vi "Initialize Millisecond Tick Timer Q.vi"(8 "error in (no error)":errorcluster, 11 "DbgTimers in":refnum<class "DbgTimers.lvclass">) -> (0 "error out":errorcluster, 3 "DbgTimers out":refnum<class "DbgTimers.lvclass">)   [LabVIEW 2017, in "DbgTimers.lvclass"]
doc: "Developed by Kevin Thompson\nkevin@thompsonengineering.net\n\nCopyright 2018-2020\nThompson Engineering, LLC"
uses:
  DbgTimers.lvclass
  DataTypes/Millsecond Tick Timer Qdata--cluster.ctl
  DataTypes/Millisecond Tick Timer--cluster.ctl
  DbgTimers.lvclass/DbgTimers.ctl
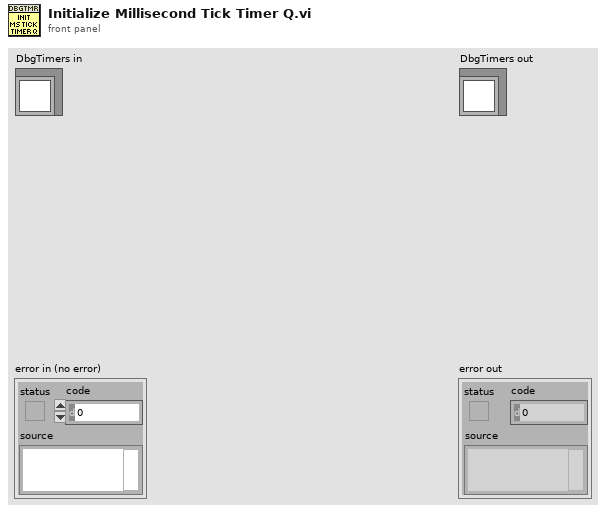
[diagram p1: front panel]
types:
  T1 = typedef "DbgTimers.lvclass/Millsecond Tick Timer Qdata--cluster.ctl" = cluster{"Time Stamp":timestamp, "comment":string, "idx":i32, "ms tick timer":T2}
  T2 = typedef "DbgTimers.lvclass/Millisecond Tick Timer--cluster.ctl" = cluster{"startTick":u32, "currentTick":u32, "elapsedTicks":u32, "totalElapsedTicks":u32}
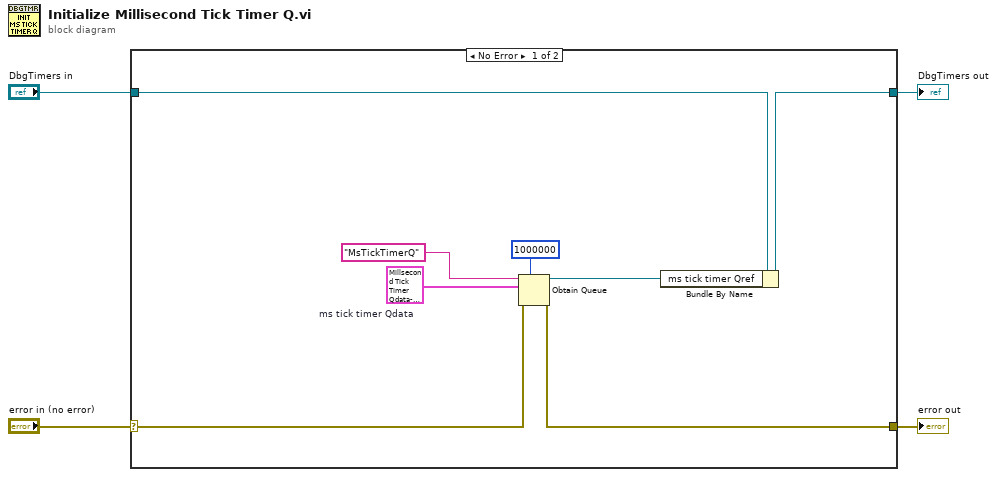
[diagram p0: block diagram]
diagram:
  n1 = case shown="No Error" "error in (no error)" {
    selector: "error in (no error)" -> [w11 w14]
    tunnel: [w10 w14] -> w3
    tunnel: [w7 w13] -> w1
    tunnel: "DbgTimers in" -> [w8 w13]
    frame No Error {
      w12 = T1 {"Time Stamp"=timestamp(0 s since 1904-01-01), "comment"="", "idx"=0, "ms tick timer"={"startTick"=0, "currentTick"=0, "elapsedTicks"=0, "totalElapsedTicks"=0}}  # ms tick timer Qdata
      n2 = Obtain Queue(max queue size (-1, unlimited)=1000000, name (unnamed)="MsTickTimerQ", element data type=w12, error in (no error)=w11) -> (queue out=w6:refnum<queue>, error out=w10:errorcluster)  [unwired: 1 in, 1 out]
      n3 = Bundle By Name(cluster=w8, "ms tick timer Qref"=w6) -> (w7:refnum<class "DbgTimers.lvclass">)
    }
    frame Error {
    }
  }
  "error out" <- w3
  "DbgTimers out" <- w1
